vi "Input Check_TextBox.vi"(8 "에러 입력":errorcluster caption="에러 입력(에러 없음)", 11 "TextBox 참조":refnum<vi>) -> (0 "에러 출력":errorcluster, 1 "Caption.Text":string, 2 "내용있음?":bool)   [LabVIEW 2020]
panel:
  out "참조 출력":refnum<vi>
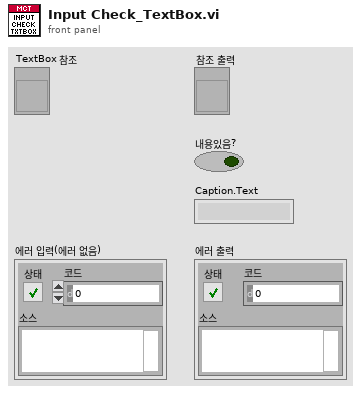
[diagram p1: front panel]
types:
  T1 = enum8{"Enabled", "Disabled", "Disabled and Grayed Out"}
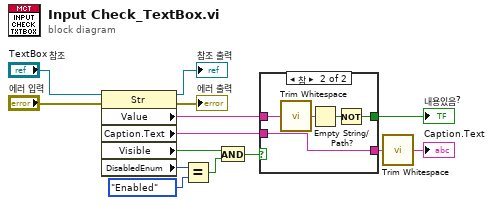
[diagram p0: block diagram]
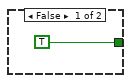
[diagram p2: hidden frame]
diagram:
  n1 = property class="Str"(reference="TextBox 참조", error in="에러 입력") -> (reference out=→"참조 출력":refnum<vi>, error out=→"에러 출력":errorcluster, "Value"=w12:string, "Caption.Text"=w11:string, "Visible"=w3:bool, "DisabledEnum"=w5:T1)
  n2 = Equal?(x=w5, y=T1."Enabled" ("비활성화")) -> (x = y?=w2:bool)
  n3 = And(x=w3, y=w2) -> (x .and. y?=w1:bool)
  n4 = case shown="참" w1 {
    tunnel: [TRUE w16] -> w14
    tunnel: w12 -> [_ w18]
    tunnel: w11 -> [_ w20]
    tunnel: [_ w20] -> w10
    frame False {
    }
    frame True {
      n5 = call <vilib>:"Trim Whitespace.vi"("string"=w18) -> ("trimmed string"=w19:string)  [unwired: 1 in]
      n6 = Empty String/Path?(string/path=w19) -> (empty?=w17:bool)
      n7 = Not(x=w17) -> (.not. x?=w16:bool)
    }
  }
  "내용있음?" <- w14
  n8 = call <vilib>:"Trim Whitespace.vi"("string"=w10) -> ("trimmed string"=→"Caption.Text":string)  [unwired: 1 in]
